vi "Read Device Channel Name.vi"(8 "error in (no error)":errorcluster, 11 "2575 in":refnum<class "2575.lvclass">) -> (0 "error out":errorcluster, 2 "Device Channel Name":T1, 3 "2575 out":refnum<class "2575.lvclass">)   [LabVIEW 2019, in "2575.lvlib" / "2575.lvclass"]
uses:
  Library/2575.lvclass
  Private/Device Channel Name.ctl
  Library/2575.lvclass/2575.ctl
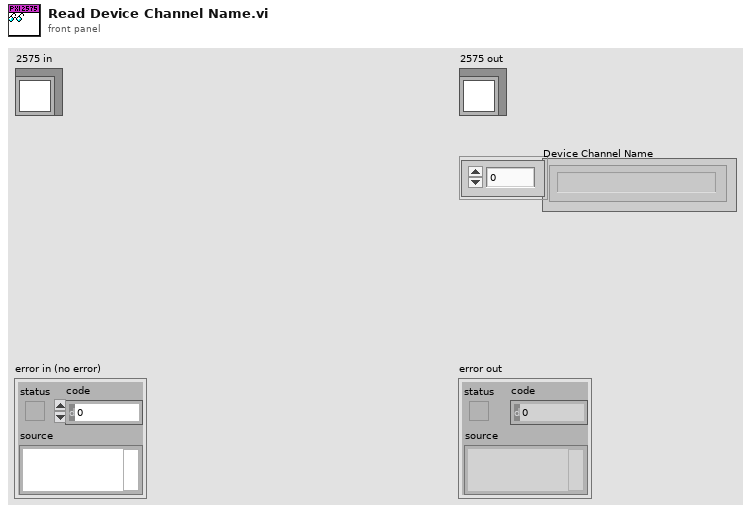
[diagram p1: front panel]
types:
  T1 = typedef "2575.lvlib/2575.lvclass/Device Channel Name.ctl" = string[]
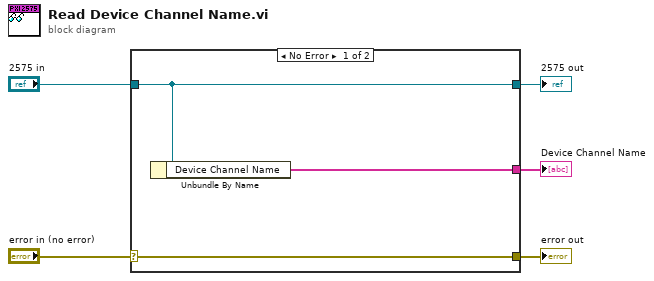
[diagram p0: block diagram]
diagram:
  n1 = case shown="No Error" "error in (no error)" {
    selector: "error in (no error)" -> [w8 w9]
    tunnel: [w8 w9] -> w4
    tunnel: [w7 w10] -> w2
    tunnel: "2575 in" -> [w7 w10]
    tunnel: [w6 _] -> w1
    frame No Error {
      n2 = Unbundle By Name(w7) -> ("Device Channel Name"=w6:string[])
    }
    frame Error {
    }
  }
  "error out" <- w4
  "2575 out" <- w2
  "Device Channel Name" <- w1
